vi "Select PPMS Class.vi"(8 "error in (no error)":errorcluster, 11 "Select PPMS":T1=enum."Simulate PPMS") -> (0 "error out":errorcluster, 3 "instrument.PPMS out":refnum<class "instrument.PPMS.lvclass">)   [LabVIEW 2019, in "PPMS.lvlib"]
uses:
  PPMS.lvlib
  instrument.PPMS/instrument.PPMS.lvclass
  Select PPMS--Enum.ctl
  instrument.PPMS1/instrument.PPMS1.lvclass
  C:/Users/patrick/Documents/GitHub/levylabpitt/PPMS-Monitor-and-Control/lvsrc/instrument.PPMS/instrument.PPMS.lvclass
  instrument.PPMS2/instrument.PPMS2.lvclass
  instrument.PPMS3/instrument.PPMS3.lvclass
  instrument.PPMS-W-1/instrument.PPMS-W-1.lvclass
  instrument.OptiCool/instrument.OptiCool.lvclass
  instrument.PPMS/instrument.PPMS.lvclass/instrument.PPMS.ctl
  C:/Program Files (x86)/National Instruments/LabVIEW 2019/user.lib/LevyLab/Instrument Framework/Instrument Types/Cryostat/Instrument.Cryostat.lvclass
  C:/Program Files (x86)/National Instruments/LabVIEW 2019/user.lib/LevyLab/Instrument Framework/Instrument/Instrument.lvclass
  C:/Program Files (x86)/National Instruments/LabVIEW 2019/vi.lib/JKI/JKI SMO/SMO/SMO.lvclass
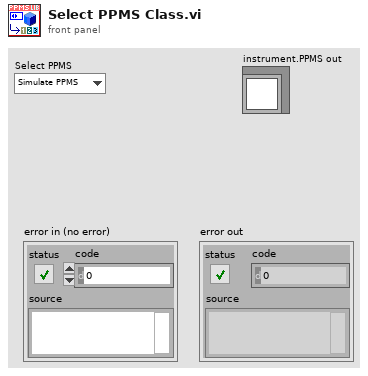
[diagram p1: front panel]
types:
  T1 = typedef "PPMS.lvlib/Select PPMS--Enum.ctl" = enum16{"PPMS1", "PPMS2", "PPMS3", "OptiCool", "PPMS-W-1", "Simulate PPMS", "Simulate DynaCool", "Simulate OptiCool"}
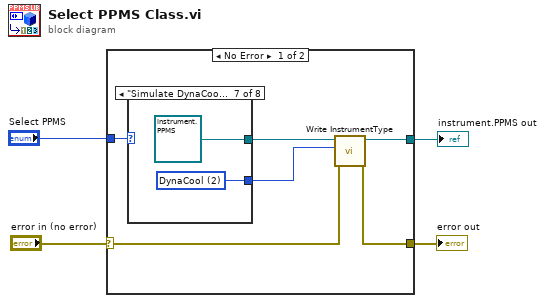
[diagram p0: block diagram]
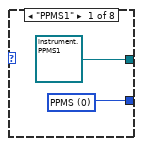
[diagram p2: hidden frame]
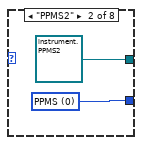
[diagram p3: hidden frame]
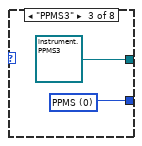
[diagram p4: hidden frame]
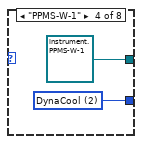
[diagram p5: hidden frame]
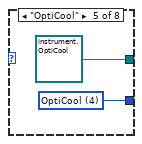
[diagram p6: hidden frame]
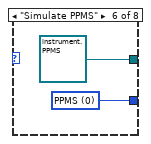
[diagram p7: hidden frame]
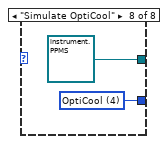
[diagram p8: hidden frame]
diagram:
  n1 = case shown="No Error" "error in (no error)" {
    selector: "error in (no error)" -> [w7 w27]
    tunnel: [w5 _] -> w4
    tunnel: "Select PPMS" -> [w10 _]
    tunnel: [w6 w27] -> w1
    frame No Error {
      n2 = case shown="\"Simulate DynaCool\"" w10 {
        tunnel: [refnum<class "instrument.PPMS1.lvclass"> refnum ("instrument.PPMS1.lvclass") refnum<class "instrument.PPMS2.lvclass"> refnum ("instrument.PPMS2.lvclass") refnum<class "instrument.PPMS3.lvclass"> refnum ("instrument.PPMS3.lvclass") refnum<class "instrument.PPMS-W-1.lvclass"> refnum ("instrument.PPMS-W-1.lvclass") refnum<class "instrument.OptiCool.lvclass"> refnum ("instrument.OptiCool.lvclass") refnum<class "instrument.PPMS.lvclass"> refnum ("instrument.PPMS2.lvclass") refnum<class "instrument.PPMS.lvclass"> refnum ("instrument.PPMS2.lvclass") refnum<class "instrument.PPMS.lvclass"> refnum ("instrument.PPMS2.lvclass")] -> w8
        tunnel: [w11 w13 w15 w18 w19 w21 w23 w25] -> w9
        frame "PPMS1" {
          w11 = 0 items=["PPMS", "VersaLab", "DynaCool", "SVSM", "OptiCool"] ("InstrumentType")
        }
        frame "PPMS2" {
          w13 = 0 items=["PPMS", "VersaLab", "DynaCool", "SVSM", "OptiCool"] ("InstrumentType")
        }
        frame "PPMS3" {
          w15 = 0 items=["PPMS", "VersaLab", "DynaCool", "SVSM", "OptiCool"] ("InstrumentType")
        }
        frame "PPMS-W-1" {
          w18 = 2 items=["PPMS", "VersaLab", "DynaCool", "SVSM", "OptiCool"] ("InstrumentType")
        }
        frame "OptiCool" {
          w19 = 4 items=["PPMS", "VersaLab", "DynaCool", "SVSM", "OptiCool"] ("InstrumentType")
        }
        frame "Simulate PPMS" {
          w21 = 0 items=["PPMS", "VersaLab", "DynaCool", "SVSM", "OptiCool"] ("InstrumentType")
        }
        frame "Simulate DynaCool" {
          w23 = 2 items=["PPMS", "VersaLab", "DynaCool", "SVSM", "OptiCool"] ("InstrumentType")
        }
        frame "Simulate OptiCool" {
          w25 = 4 items=["PPMS", "VersaLab", "DynaCool", "SVSM", "OptiCool"] ("InstrumentType")
        }
      }
      n3 = call "Write InstrumentType.vi"("error in (no error)"=w7, "InstrumentType"=w9, "instrument.PPMS in"=w8) -> ("error out"=w6:errorcluster, "instrument.PPMS out"=w5:refnum<class "instrument.PPMS.lvclass">)  [unwired: 7 in]
    }
    frame Error {
    }
  }
  "instrument.PPMS out" <- w4
  "error out" <- w1
